vi "Init.vi"(8 "error in (no error)":errorcluster, 11 "Serial Devices in":refnum<class "Serial Devices.lvclass">) -> (0 "error out":errorcluster, 3 "Serial Devices out":refnum<class "Serial Devices.lvclass">)   [LabVIEW 2019, in "Serial Devices.lvlib" / "Serial Devices.lvclass"]
uses:
  Serial Devices.lvclass
  C:/Program Files (x86)/National Instruments/LabVIEW 2019/vi.lib/ActorFramework/Actor/Actor.lvclass
  <vilib>/ActorFramework/Actor/Actor.lvclass/Actor.ctl
  <vilib>/ActorFramework/Message Enqueuer/Message Enqueuer.lvclass/Message Enqueuer.ctl
  Serial Devices.lvclass/Serial Devices.ctl
  NXP/NXP.lvclass
  NXP/NXP.lvclass/NXP.ctl
  TI/CYPRESS.lvclass
  TI/CYPRESS.lvclass/CYPRESS.ctl
  SIMULATED/SIMULATED.lvclass
  SIMULATED/SIMULATED.lvclass/SIMULATED.ctl
  NXP/Write COM SELECTED NXP.vi
  NXP/Write SIMULATED_ NXP.vi
  Read BRAND SELECTED.vi
  Read COM SELECTED.vi
  Read SIMULATED_.vi
  Read This VI.vi
  <vilib>/ActorFramework/Message Enqueuer/Init from Existing Queue.vi
  <vilib>/ActorFramework/Message Enqueuer/Message Enqueuer.lvclass
  <vilib>/ActorFramework/Actor/Actor.lvclass
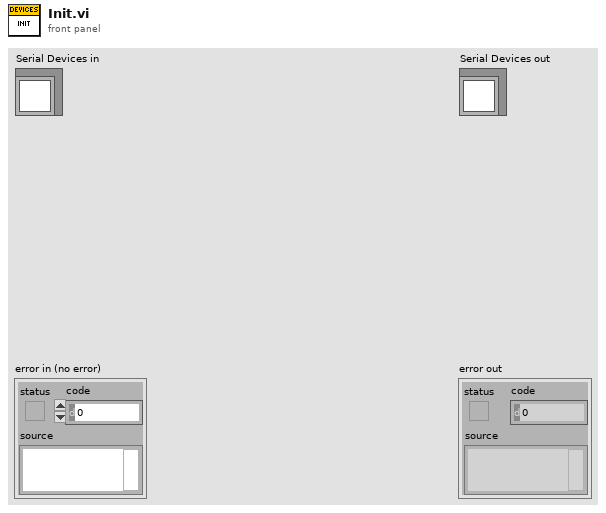
[diagram p1: front panel]
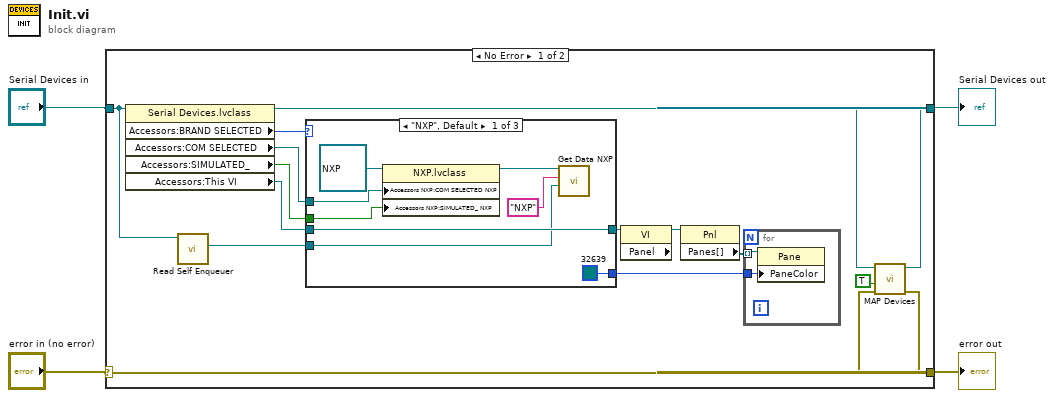
[diagram p0: block diagram]
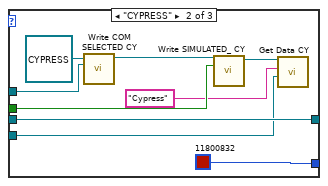
[diagram p2: hidden frame]
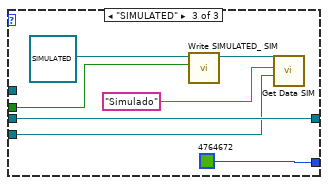
[diagram p3: hidden frame]
diagram:
  n1 = case shown="No Error" "error in (no error)" {
    selector: "error in (no error)" -> [w8 w47]
    tunnel: [w7 w47] -> w1
    tunnel: [w6 w46] -> w2
    tunnel: "Serial Devices in" -> [w11 w46]
    frame No Error {
      n2 = property class="Serial Devices.lvclass"(reference=w11) -> (reference out=w9:refnum<class "Serial Devices.lvclass">, "Accessors:BRAND SELECTED"=w19:enum16{"NXP", "CYPRESS", "SIMULATED"}, "Accessors:COM SELECTED"=w17:refnum<visa-resource-name>, "Accessors:SIMULATED_"=w18:bool, "Accessors:This VI"=w16:refnum<vi>)  [unwired: 1 in, 1 out]
      n3 = call <vilib>:"Read Self Enqueuer.vi"("Actor"=w11) -> ("Self Enqueuer"=w10:refnum<class "Message Enqueuer.lvclass">)  [unwired: 10 in]
      n4 = case shown="\"NXP\", Default" w19 {
        tunnel: w18 -> [w23 w33 w45]
        tunnel: w17 -> [w24 w35 _]
        tunnel: w16 -> [w28 w38 w42]
        tunnel: [w28 w38 w42] -> w15
        tunnel: [u32 32639 u32 11800832 u32 4764672] -> w12
        tunnel: w10 -> [w26 w31 w40]
        frame "NXP", Default {
          n5 = property class="NXP.lvclass"(reference=refnum<class "NXP.lvclass"> refnum ("NXP.lvclass"), "Accessors NXP:COM SELECTED NXP"=w24, "Accessors NXP:SIMULATED_ NXP"=w23) -> (reference out=w22:refnum<class "NXP.lvclass">)  [unwired: 1 in, 1 out]
          n6 = call "Get Data NXP.vi"("Data Enqueuer"=w26, "Data"="NXP", "NXP in"=w22) -> ()  [unwired: 7 in, 2 out]
        }
        frame "CYPRESS" {
          n7 = call "Write COM SELECTED CY.vi"("COM SELECTED"=w35, "TI in"=refnum<class "CYPRESS.lvclass"> refnum ("CYPRESS.lvclass")) -> ("TI out"=w34:refnum<class "CYPRESS.lvclass">)  [unwired: 8 in, 1 out]
          n8 = call "Write SIMULATED_ CY.vi"("SIMULATED?"=w33, "TI in"=w34) -> ("TI out"=w32:refnum<class "CYPRESS.lvclass">)  [unwired: 8 in, 1 out]
          n9 = call "Get Data CY.vi"("Data Enqueuer"=w31, "Data"="Cypress", "CYPRESS in"=w32) -> ()  [unwired: 7 in, 2 out]
        }
        frame "SIMULATED" {
          n10 = call "Write SIMULATED_ SIM.vi"("SIMULATED?"=w45, "SIMULATED in"=refnum<class "SIMULATED.lvclass"> refnum ("SIMULATED.lvclass")) -> ("SIMULATED out"=w41:refnum<class "SIMULATED.lvclass">)  [unwired: 8 in, 1 out]
          n11 = call "Get Data SIM.vi"("Data Enqueuer"=w40, "Data"="Simulado", "SIMULATED in"=w41) -> ()  [unwired: 7 in, 2 out]
        }
      }
      n12 = property class="VI"(reference=w15) -> ("Panel"=w14:refnum<vi>)  [unwired: 1 in, 2 out]
      n13 = property class="Pnl"(reference=w14) -> ("Panes[]"=w13:refnum<vi>[])  [unwired: 1 in, 2 out]
      n14 = for {
        tunnel: w13 -> [w21] mode=indexing
        tunnel: w12 -> [w20]
        n15 = property class="Pane"(reference=w21, "PaneColor"=w20) -> ()  [unwired: 1 in, 2 out]
      }
      n16 = call "MAP Devices.vi"("error in (no error)"=w8, "CREAR"=TRUE, "Serial Devices in"=w9) -> ("error out"=w7:errorcluster, "Serial Devices out"=w6:refnum<class "Serial Devices.lvclass">)  [unwired: 6 in, 1 out]
    }
    frame Error {
    }
  }
  "error out" <- w1
  "Serial Devices out" <- w2
